vi "Cannon Get.vi"(0 "Shoot!":T1) -> ()   [LabVIEW 2013]
uses:
  <vilib>/Rock Robotics/WPI/Solenoid/WPI_SolenoidValue.ctl
  Cannon Global Data.vi
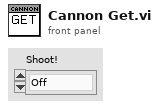
[diagram p1: front panel]
types:
  T1 = typedef "WPI_SolenoidValue.ctl" = enum16{"Off", "On", "Forward", "Reverse"}
  T2 = typedef "WPI_DigitalInputDevRef.ctl" = cluster{"DevStatus":errorcluster, "DIO Channel":T3, "Digital Module":T4}
  T3 = typedef "FPGA_DIOChannel.ctl" = enum8{"DIO 1", "DIO 2", "DIO 3", "DIO 4", "DIO 5", "DIO 6", "DIO 7", "DIO 8", "DIO 9", "DIO 10", "DIO 11", "DIO 12", "DIO 13", "DIO 14", "Invalid"}
  T4 = typedef "FPGA_TypedefDigitalModule.ctl" = enum16{"Digital Module 1", "Digital Module 2"}
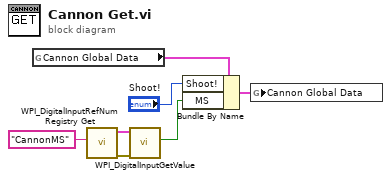
[diagram p0: block diagram]
diagram:
  n1 = global read "Cannon Global Data.vi" "Cannon Global Data"() -> (w2:cluster{"MS":bool, "Shoot!":T1})
  n2 = call <vilib>:"WPI_DigitalInputRefNum Registry Get.vi"("refnum name"="CannonMS") -> ("error out"=w4:errorcluster, "DigitalInputDevRef"=w5:T2)  [unwired: 9 in]
  n3 = call <vilib>:"WPI_DigitalInputGetValue.vi"("error in (no error)"=w4, "DigitalInputDevRef"=w5) -> ("Value"=w6:bool)  [unwired: 7 in, 2 out]
  n4 = Bundle By Name(cluster=w2, "Shoot!"="Shoot!", "MS"=w6) -> (w1:cluster{"MS":bool, "Shoot!":T1})
  n5 = global write "Cannon Global Data.vi" "Cannon Global Data"(w1) -> ()
